vi "Write and Read Multiple Holding Registers.vi"(4 "read count":u16, 6 "read starting address":u16, 7 "unit ID":u8, 8 "error in":errorcluster, 9 "write values":u16[](array[numeric]), 10 "write starting address":u16, 11 "Modbus instance in":refnum<class "Modbus Master.lvclass">) -> (0 "error out":errorcluster, 1 "read values":u16[](array[numeric]), 3 "Modbus instance out":refnum<class "Modbus Master.lvclass">)   [LabVIEW 2013, in "Modbus Library - Advance.lvlib" / "Modbus Master.lvclass"]
doc: "Writes and reads the values of multiple register values in series. The <b>write values</b> are inserted starting at <b>write starting address</b> and the returned <b>read values</b> consists of <b>read count</b> holding registers starting at <b>read starting address</b>."
uses:
  Modbus Master.lvclass
  Modbus Master.lvclass/Modbus Master.ctl
  Modbus API.lvclass/Modbus API.ctl
  Transmission Data Unit/Transmission Data Unit.lvclass/Transmission Data Unit.ctl
  Transmission Data Unit/Transmission Data Unit.lvclass
  Master Function Definition/Master Function Definition.lvclass
  Modbus API.lvclass
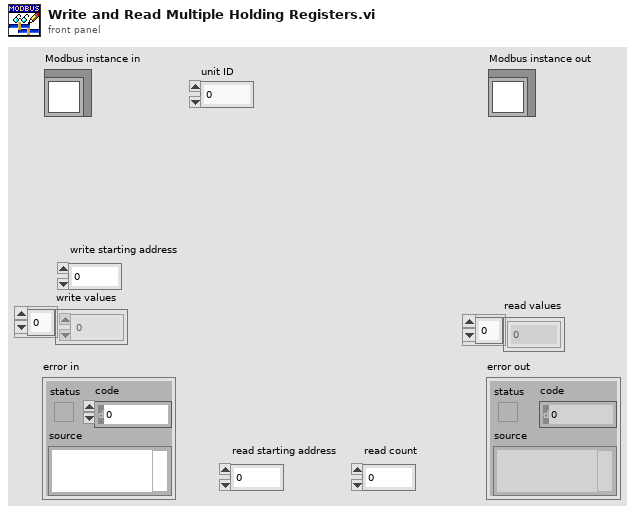
[diagram p1: front panel]
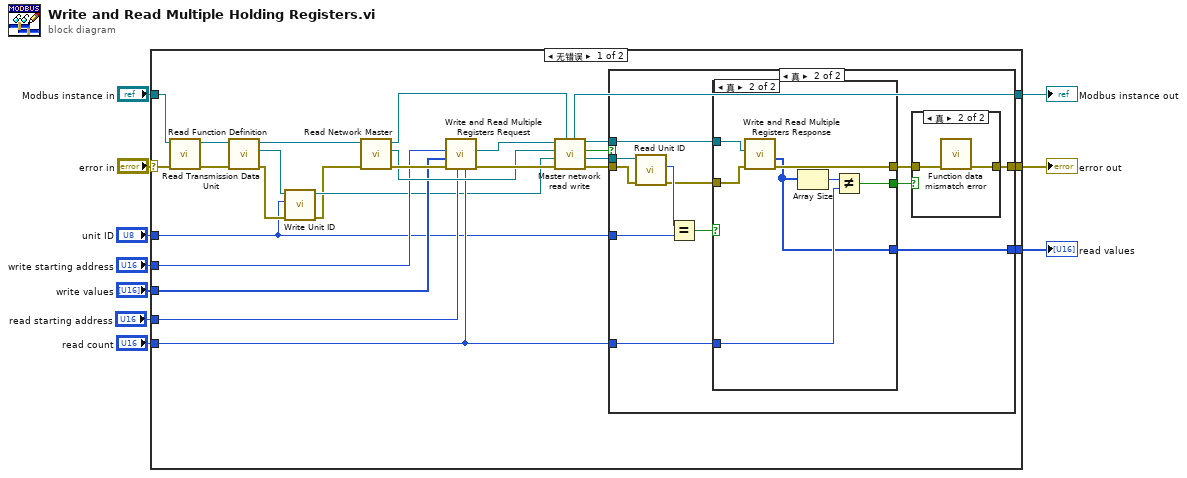
[diagram p0: block diagram]
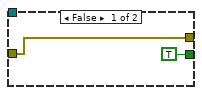
[diagram p3: hidden frame]
diagram:
  n1 = case shown="无错误" "error in" {
    selector: "error in" -> [w27 w62]
    tunnel: "Modbus instance in" -> [w25 w63]
    tunnel: [w31 w63] -> w9
    tunnel: [w35 w62] -> w8
    tunnel: "read count" -> [w22 _]
    tunnel: [w21 _] -> w5
    tunnel: "read starting address" -> [w20 _]
    tunnel: "write values" -> [w19 _]
    tunnel: "write starting address" -> [w18 _]
    tunnel: "unit ID" -> [w11 _]
    frame No Error {
      n2 = call "Read Function Definition.vi"("error in"=w27, "Modbus master in"=w25) -> ("error out"=w29:errorcluster, "Modbus master out"=w28:refnum<class "Modbus Master.lvclass">)  [unwired: 7 in, 1 out]
      n3 = call "Read Transmission Data Unit.vi"("error in"=w29, "Modbus instance in"=w28) -> ("error out"=w13:errorcluster, "transmission data unit"=w15:refnum<class "Transmission Data Unit.lvclass">, "Modbus instance out"=w30:refnum<class "Modbus Master.lvclass">)  [unwired: 7 in]
      n4 = call "Write Unit ID.vi"("error in"=w13, "unit ID"=w11, "transmission data unit in"=w15) -> ("error out"=w12:errorcluster, "transmission data unit out"=w14:refnum<class "Transmission Data Unit.lvclass">)  [unwired: 7 in]
      n5 = call "Read Network Master.vi"("error in"=w12, "Modbus master in"=w30) -> ("error out"=w26:errorcluster, "network master"=w23:refnum<class "Network Master.lvclass">, "Modbus master out"=w24:refnum<class "Modbus Master.lvclass">)  [unwired: 7 in]
      n6 = call "Write and Read Multiple Registers Request.vi"("Quantity to Read"=w22, "Read Starting Address"=w20, "error in"=w26, "Write"=w19, "Write Starting Address"=w18) -> ("error out"=w36:errorcluster, "modbus data unit out"=w33:refnum<class "Modbus Data Unit.lvclass">)  [unwired: 5 in]
      n7 = call "Master network read write.vi"("Modbus master in"=w24, "error in"=w36, "transmission data unit in"=w14, "network master in"=w23, "Modbus data unit in"=w33) -> ("error out"=w34:errorcluster, "transmission data unit out"=w16:refnum<class "Transmission Data Unit.lvclass">, "PDU Valid?"=w17:bool, "Modbus data unit out"=w32:refnum<class "Modbus Data Unit.lvclass">, "Modbus master out"=w31:refnum<class "Modbus Master.lvclass">)  [unwired: 2 in]
      n8 = case shown="真" w17 {
        tunnel: [w37 w49] -> w35
        tunnel: w34 -> [w37 w42]
        tunnel: w32 -> [_ w48]
        tunnel: w22 -> [_ w45]
        tunnel: [_ w44] -> w21
        tunnel: w16 -> [_ w43]
        tunnel: w11 -> [_ w40]
        frame False {
        }
        frame True {
          n9 = call "Read Unit ID.vi"("error in"=w42, "transmission data unit in"=w43) -> ("error out"=w38:errorcluster, "unit ID"=w41:u8)  [unwired: 7 in, 1 out]
          n10 = Equal?(x=w41, y=w40) -> (x = y?=w39:bool)
          n11 = case shown="真" w39 {
            tunnel: w48 -> [_ w58]
            tunnel: [w51 w57] -> w47
            tunnel: [TRUE w56] -> w46
            tunnel: w45 -> [_ w54]
            tunnel: [_ w53] -> w44
            tunnel: w38 -> [w51 w52]
            frame False {
            }
            frame True {
              n12 = call "Write and Read Multiple Registers Response.vi"("error in"=w52, "modbus data unit in"=w58) -> ("error out"=w57:errorcluster, "Registers"=w53:u16[])  [unwired: 7 in, 1 out]
              n13 = Array Size(array=w53) -> (size(s)=w55:i32)
              n14 = Not Equal?(x=w55, y=w54) -> (x != y?=w56:bool)
            }
          }
          n15 = case shown="真" w46 {
            tunnel: [w59 w61] -> w49
            tunnel: w47 -> [w59 w60]
            frame False {
            }
            frame True {
              n16 = call "Function data mismatch error.vi"("error in (no error)"=w60) -> ("error out"=w61:errorcluster)  [unwired: 10 in]
            }
          }
        }
      }
    }
    frame Error {
    }
  }
  "error out" <- w8
  "Modbus instance out" <- w9
  "read values" <- w5
